vi "Pull_Data_Client.vi"(1 "Running on Server?":bool, 2 "application reference":refnum<vi>, 3 "error in (no error)":errorcluster, 4 "File to Archive":path[](array[path]), 5 "Files to Pull":path[](array[path]), 6 "Relative Path":path=path "/Lacie_20/test") -> (0 "error out":errorcluster)   [LabVIEW 2011]
uses:
  Anemometry/Anemometry Sub Vis/Globals/Constants_global.vi
  <vilib>/zip/NI_Unzip.lvlib
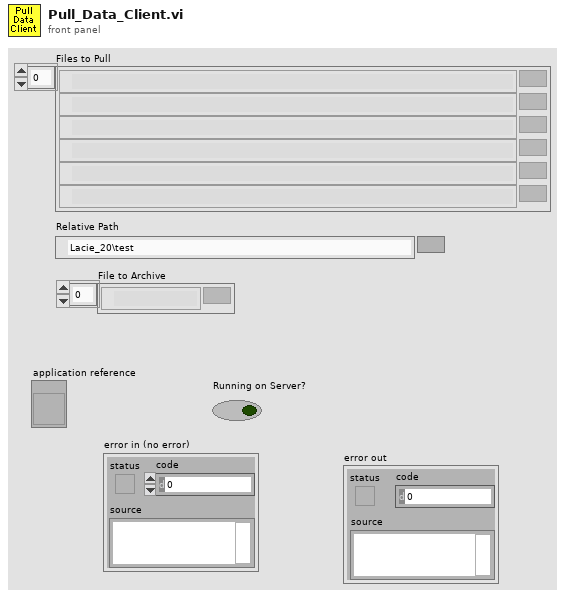
[diagram p1: front panel]
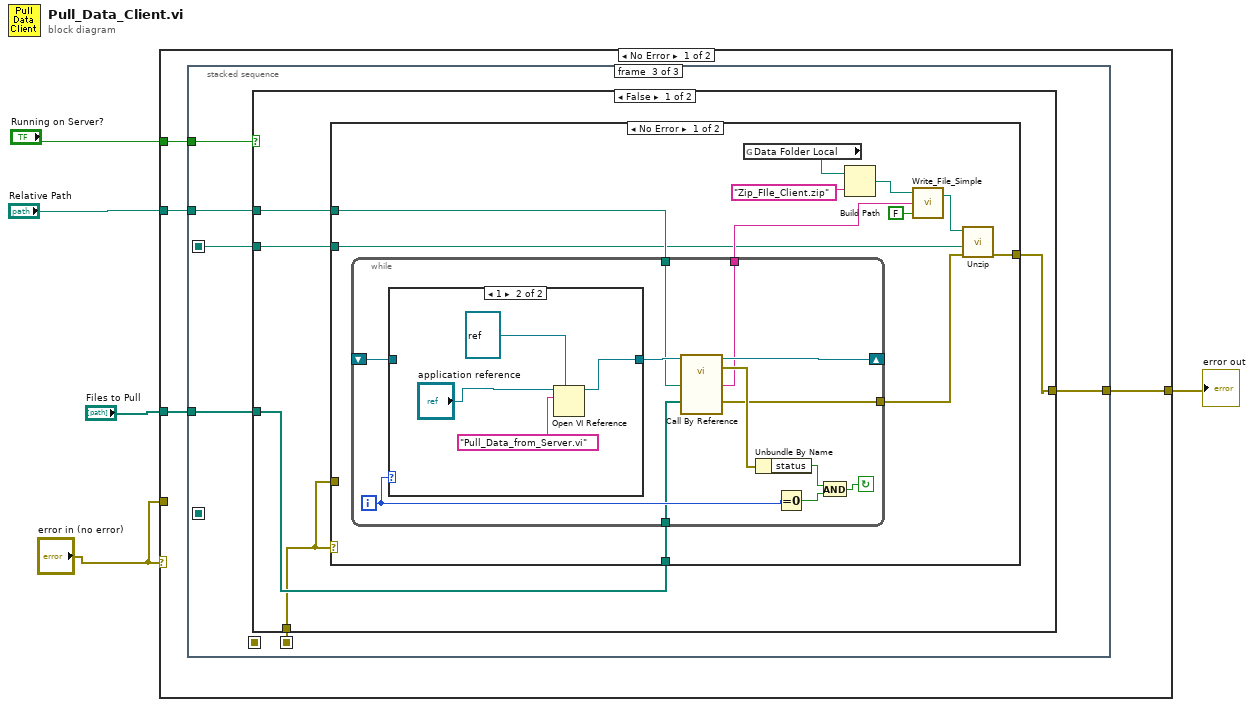
[diagram p0: block diagram]
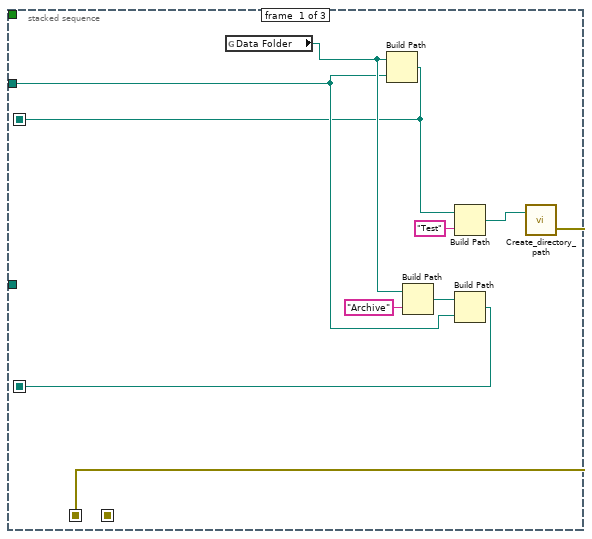
[diagram p2: hidden frame]
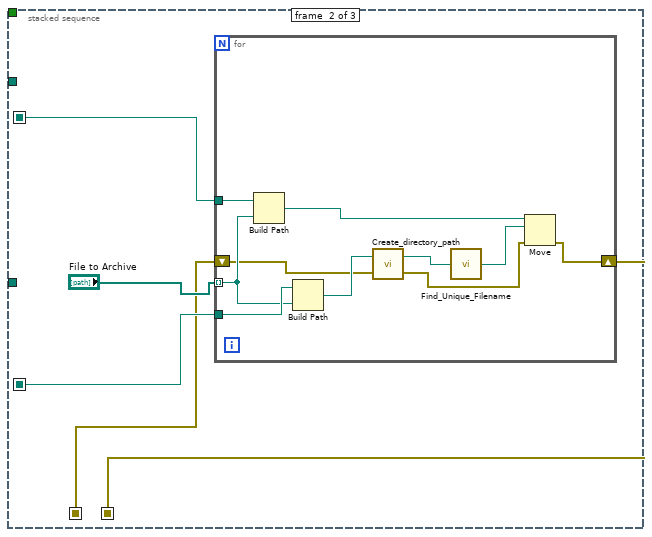
[diagram p3: hidden frame]
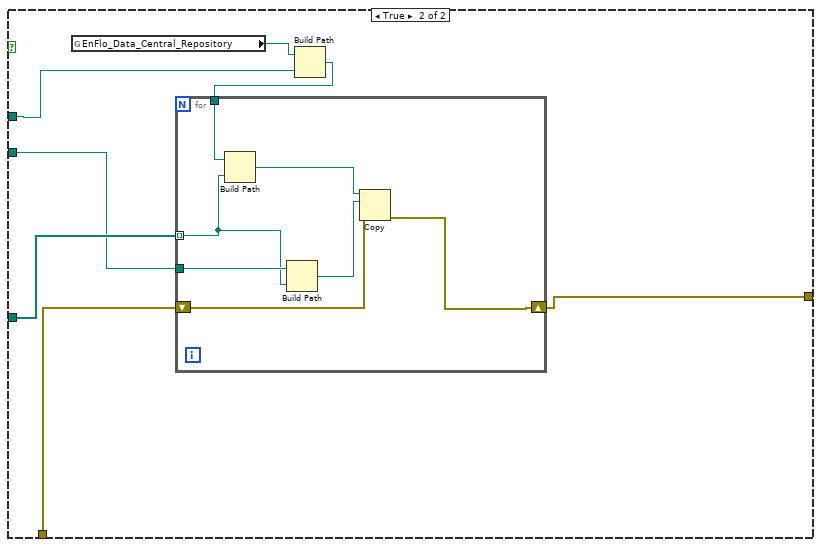
[diagram p6: hidden frame]
diagram:
  n1 = case shown="No Error" "error in (no error)" {
    tunnel: "Relative Path" -> [w9 _]
    tunnel: "Files to Pull" -> [w8 _]
    tunnel: "Running on Server?" -> [w7 _]
    tunnel: [w6 w88] -> w2
    tunnel: "error in (no error)" -> [_ w88]
    frame No Error {
      n2 = stacked-sequence {
        seq-local: [w12 _ _] -> [_ w21 w37]
        seq-local: [w11 _ _] -> [_ w23 _]
        seq-local: [w10 _ _] -> [_ w20 _]
        seq-local: [_ w19 _] -> [_ _ w34]
        tunnel: w9 -> [w13 _ w39]
        tunnel: w8 -> [_ _ w38]
        tunnel: w7 -> [_ _ w36]
        tunnel: [_ _ w35] -> w6
        frame #0 {
          n3 = global read "Constants_global.vi" "Data Folder"() -> (w14:path)
          n4 = Build Path(base path=w14, name or relative path=w13) -> (appended path=w12:path)
          n5 = Build Path(base path=w14, name or relative path="Archive") -> (appended path=w18:path)
          n6 = Build Path(base path=w12, name or relative path="Test") -> (appended path=w15:path)
          n7 = Build Path(base path=w18, name or relative path=w13) -> (appended path=w11:path)
          n8 = call "Create_directory_path.vi"("Path name"=w15) -> ("error out"=w10:errorcluster)  [unwired: 1 in, 1 out]
        }
        frame #1 {
          n9 = for {
            tunnel: w21 -> [w33]
            tunnel: "File to Archive" -> [w30] mode=indexing
            tunnel: w23 -> [w31]
            shift-right: [w26] -> w19
            shift-left: w20 -> [w25]
            n10 = Build Path(base path=w33, name or relative path=w30) -> (appended path=w32:path)
            n11 = Build Path(base path=w31, name or relative path=w30) -> (appended path=w28:path)
            n12 = call "Create_directory_path.vi"("error in (no error)"=w25, "Path name"=w28) -> ("error out"=w24:errorcluster, "Path name Out"=w27:path)
            n13 = call "Find_Unique_Filename.vi"("Path In"=w27) -> ("Unique Path Out"=w29:path)  [unwired: 2 in]
            n14 = Move(source path=w32, error in=w24, 10:w29) -> (error out=w26:errorcluster)  [unwired: 2 in, 2 out]
          }
        }
        frame #2 {
          n15 = case shown="False" w36 {
            tunnel: w39 -> [w44 w78]
            tunnel: w38 -> [w43 w80]
            tunnel: w37 -> [w42 w76]
            tunnel: [w41 w75] -> w35
            tunnel: w34 -> [w40 w74]
            frame False {
              n16 = case shown="No Error" w40 {
                tunnel: w44 -> [w55 _]
                tunnel: w43 -> [w54 _]
                tunnel: w42 -> [w47 _]
                tunnel: [w45 w73] -> w41
                tunnel: w40 -> [_ w73]
                frame No Error {
                  n17 = while {
                    shift-right: [w65] -> _
                    shift-left: _ -> [w67]
                    tunnel: w55 -> [w59]
                    tunnel: w54 -> [w58]
                    tunnel: [w57] -> w48
                    tunnel: [w56] -> w46
                    i -> [w63]
                    stop <- w60 continue-if-true
                    n18 = case shown="1" w63 {
                      tunnel: w67 -> [w68 _]
                      tunnel: [w68 w72] -> w66
                      frame 0, Default {
                      }
                      frame 1 {
                        n19 = Open VI Reference(type specifier VI Refnum (for type only)=refnum<vi> refnum ("Push Data Server"), application reference (local)="application reference", vi path="Pull_Data_from_Server.vi") -> (vi reference=w72:refnum<vi>)  [unwired: 1 in, 3 out]
                      }
                    }
                    n20 = call-by-ref "?"(reference=w66, "Files to Pull"=w58, "Relative Path"=w59) -> (reference out=w65:refnum<vi>, error out=w64:errorcluster, "error out"=w56:errorcluster, "Zip File String"=w57:string)  [unwired: 1 in]
                    n21 = Unbundle By Name(w64) -> ("status"=w61:bool)
                    n22 = Equal To 0?(x=w63) -> (x = 0?=w62:bool)
                    n23 = And(x=w61, y=w62) -> (x .and. y?=w60:bool)
                  }
                  n24 = global read "Constants_global.vi" "Data Folder Local"() -> (w50:path)
                  n25 = Build Path(base path=w50, name or relative path="Zip_FIle_Client.zip") -> (appended path=w49:path)
                  n26 = call "Write_File_Simple.vi"("append to file? (new file:F)"=FALSE, "character string"=w48, "file path"=w49) -> ("file path Out"=w53:path)  [unwired: 1 out]
                  n27 = call <vilib>:"Unzip.vi"("error in (no error)"=w46, "Target directory (same as Zip file if empty)"=w47, "Zip file"=w53) -> ("error out"=w45:errorcluster)  [unwired: 6 in, 2 out]
                }
                frame Error {
                }
              }
            }
            frame True {
              n28 = global read "Constants_global.vi" "EnFlo_Data_Central_Repository"() -> (w79:path)
              n29 = Build Path(base path=w79, name or relative path=w78) -> (appended path=w77:path)
              n30 = for {
                tunnel: w80 -> [w86] mode=indexing
                tunnel: w76 -> [w87]
                tunnel: w77 -> [w83]
                shift-right: [w81] -> w75
                shift-left: w74 -> [w82]
                n31 = Build Path(base path=w83, name or relative path=w86) -> (appended path=w84:path)
                n32 = Build Path(base path=w87, name or relative path=w86) -> (appended path=w85:path)
                n33 = Copy(8:w82, 10:w85, 11:w84) -> (0:w81:errorcluster)  [unwired: 2 in, 2 out]
              }
            }
          }
        }
      }
    }
    frame Error {
    }
  }
  "error out" <- w2
